vi "Run.vi"(4 "Boolean":bool, 6 "Numeric":dbl, 8 "error in (no error)":errorcluster, 9 "Assembly Type":string, 10 "Control In":T1={"I-O.lvclass"=refnum, "Gantry"=refnum, "Dispenser"="COM1"}, 11 "Assembly In":refnum<class "Calibrate.lvclass">) -> (0 "error out":errorcluster, 2 "Control Out":T1={"I-O.lvclass"=refnum, "Gantry"=refnum, "Dispenser"="COM1"}, 3 "Assembly Out":refnum<class "Calibrate.lvclass">)   [LabVIEW 2021, in "Calibrate.lvclass"]
uses:
  Calibrate.lvclass
  Controller/Controllers.ctl
  Controller/I-O/I-O.lvclass
  C:/Program Files (x86)/Aerotech/A3200/LabVIEW/2010/Bin/Aerotech.A3200.dll
  Program Files (x86)/Aerotech/A3200/LabVIEW/2010/Bin/Aerotech.A3200.dll
  Calibrate.lvclass/Calibrate.ctl
  Assembly Run.lvclass
  Module/Module.lvclass
  Controller/Controller.lvclass
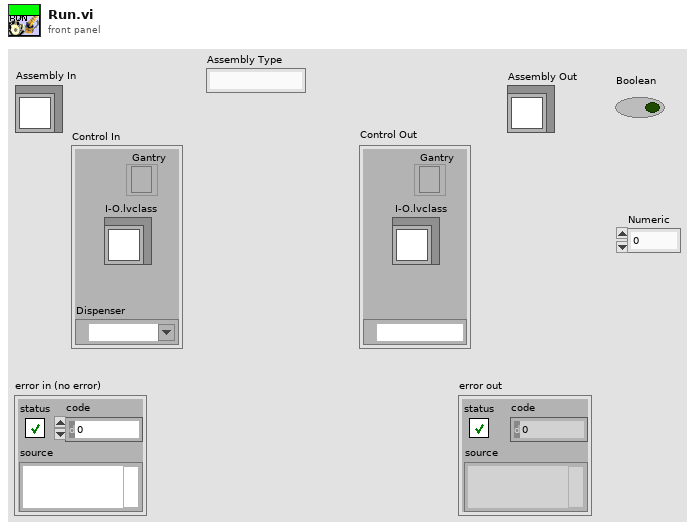
[diagram p1: front panel]
types:
  T1 = typedef "Controller.lvclass/Controllers.ctl" = cluster{"I-O.lvclass":refnum<class "I-O.lvclass">, "Gantry":refnum<k24>, "Dispenser":refnum<visa-resource-name>}
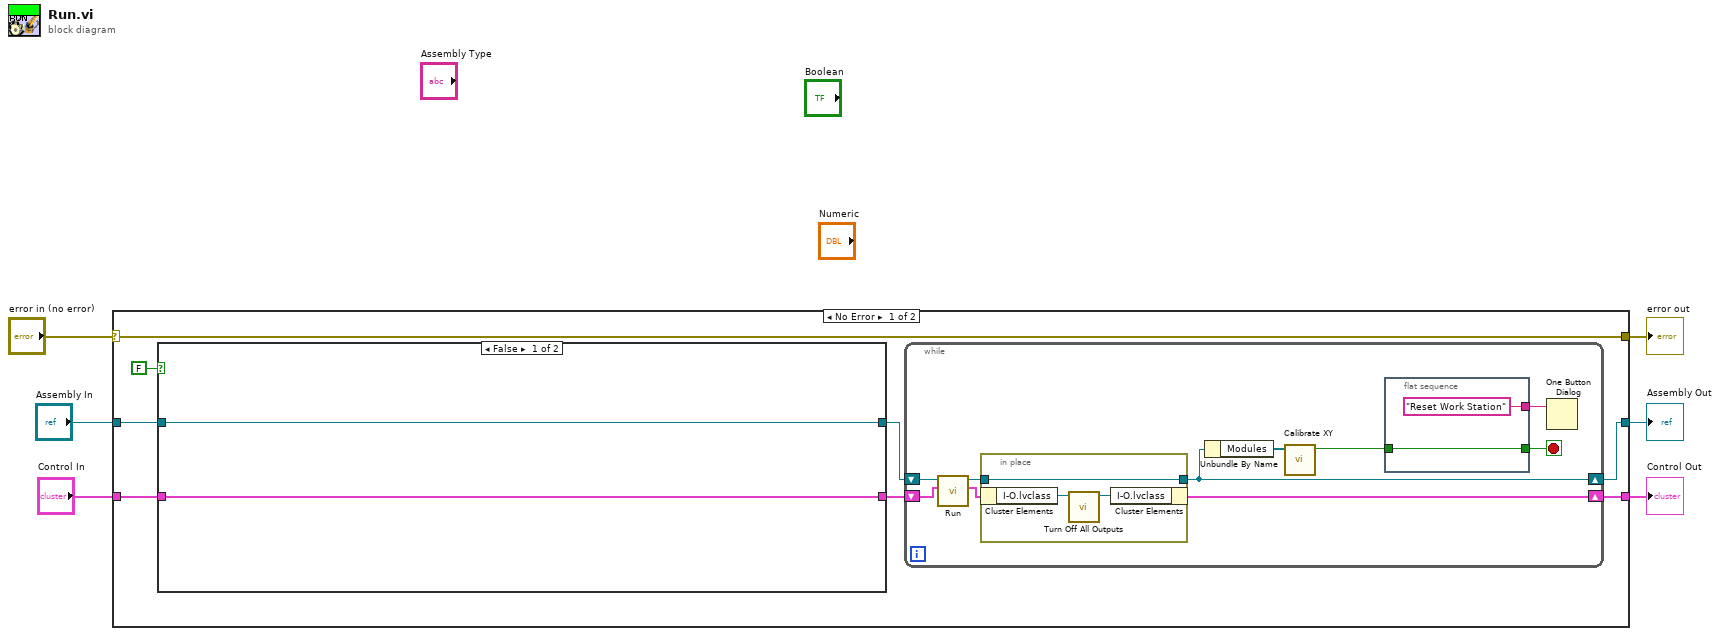
[diagram p0: block diagram]
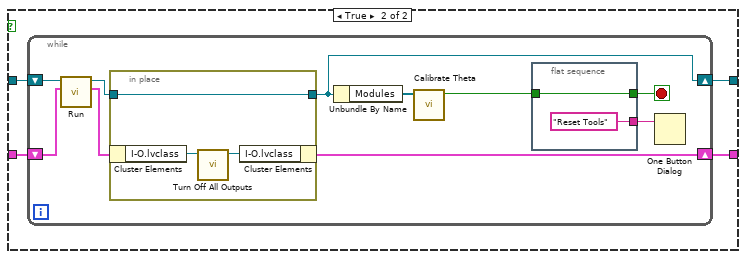
[diagram p2: hidden frame]
diagram:
  n1 = case shown="No Error" "error in (no error)" {
    selector: "error in (no error)" -> [w8 w53]
    tunnel: "Control In" -> [w14 w51]
    tunnel: "Assembly In" -> [w12 w52]
    tunnel: [w11 w51] -> w4
    tunnel: [w9 w52] -> w3
    tunnel: [w8 w53] -> w1
    frame No Error {
      n2 = case shown="False" FALSE {
        tunnel: w14 -> [w15 w20]
        tunnel: [w15 w19] -> w13
        tunnel: w12 -> [w16 w18]
        tunnel: [w16 w17] -> w10
        frame False {
        }
        frame True {
          n3 = while {
            shift-right: [w24] -> w19
            shift-left: w20 -> [w30]
            shift-right: [w21] -> w17
            shift-left: w18 -> [w29]
            stop <- w22 stop-if-true
            n4 = call-parent "Run.vi"("Control In"=w30, "Assembly In"=w29) -> ("Control Out"=w26:T1, "Assembly Out"=w25:refnum<class "Calibrate.lvclass">)  [unwired: 7 in, 1 out]
            n5 = in-place {
              in-place-border: w25 -> [w31]
              in-place-border: [w31] -> w21
              n6 = in-place-cluster #1(w26) -> ("I-O.lvclass"=w33:refnum<class "I-O.lvclass">)
              n7 = call-dynamic "Turn Off All Outputs.vi"("I-O in"=w33) -> ("I-O out"=w32:refnum<class "I-O.lvclass">)  [unwired: 9 in, 1 out]
              n8 = in-place-cluster #1("I-O.lvclass"=w32) -> (w24:T1)
            }
            n9 = Unbundle By Name(w21) -> ("Modules"=w28:refnum<class "Module.lvclass">[])
            n10 = call "Calibrate Theta.vi"("Modules"=w28) -> ("Continue?"=w23:bool)  [unwired: 10 in]
            n11 = flat-sequence {
              tunnel: ["Reset Tools"] -> w27
              tunnel: w23 -> [w34]
              tunnel: [w34] -> w22
              frame #0 {
              }
            }
            n12 = One Button Dialog(message=w27) -> ()  [unwired: 1 in, 1 out]
          }
        }
      }
      n13 = while {
        shift-right: [w36] -> w11
        shift-left: w13 -> [w44]
        shift-right: [w37] -> w9
        shift-left: w10 -> [w45]
        stop <- w40 stop-if-true
        n14 = call-parent "Run.vi"("Control In"=w44, "Assembly In"=w45) -> ("Control Out"=w39:T1, "Assembly Out"=w38:refnum<class "Calibrate.lvclass">)  [unwired: 7 in, 1 out]
        n15 = in-place {
          in-place-border: w38 -> [w46]
          in-place-border: [w46] -> w37
          n16 = in-place-cluster #2(w39) -> ("I-O.lvclass"=w48:refnum<class "I-O.lvclass">)
          n17 = call-dynamic "Turn Off All Outputs.vi"("I-O in"=w48) -> ("I-O out"=w47:refnum<class "I-O.lvclass">)  [unwired: 9 in, 1 out]
          n18 = in-place-cluster #2("I-O.lvclass"=w47) -> (w36:T1)
        }
        n19 = Unbundle By Name(w37) -> ("Modules"=w43:refnum<class "Module.lvclass">[])
        n20 = call "Calibrate XY.vi"("Modules"=w43) -> ("Continue?"=w41:bool)  [unwired: 10 in]
        n21 = flat-sequence {
          tunnel: ["Reset Work Station"] -> w42
          tunnel: w41 -> [w49]
          tunnel: [w49] -> w40
          frame #0 {
          }
        }
        n22 = One Button Dialog(message=w42) -> ()  [unwired: 1 in, 1 out]
      }
    }
    frame Error {
    }
  }
  "error out" <- w1
  "Control Out" <- w4
  "Assembly Out" <- w3
